vi "Trim_log.vi"(8 "error in (no error)":errorcluster, 9 "% to trim":i32=75 caption="% to trim (75)", 11 "Log File Refnum":refnum<file>) -> (0 "error out":errorcluster, 3 "Log File Refnum (out)":refnum<file>)   [LabVIEW 2010, in "lib1299.lvlib"]
uses:
  lib1299.lvlib
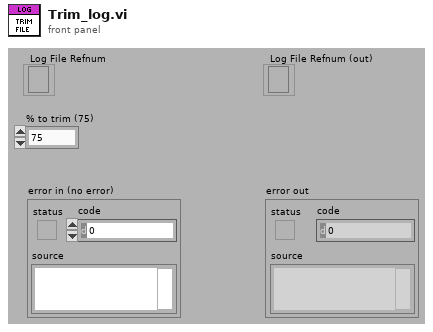
[diagram p1: front panel]
types:
  T1 = enum16{"open", "replace", "create", "open or create", "replace or create", "replace or create with confirmation"}
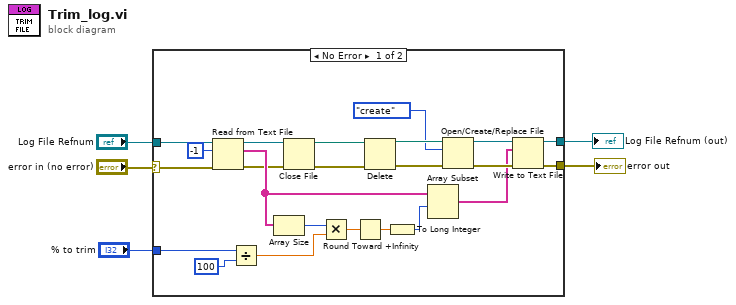
[diagram p0: block diagram]
diagram:
  n1 = case shown="No Error" "error in (no error)" {
    selector: "error in (no error)" -> [w7 w29]
    tunnel: "% to trim" -> [w25 _]
    tunnel: "Log File Refnum" -> [w19 w30]
    tunnel: [w8 w30] -> w3
    tunnel: [w6 w29] -> w1
    frame No Error {
      n2 = Read from Text File(file (use dialog)=w19, count=-1, error in=w7) -> (refnum out=w17:refnum<file>, text=w24:string[], error out=w18:errorcluster)  [unwired: 1 in, 1 out]
      n3 = Divide(x=w25, y=100 ("x")) -> (x/y=w21:dbl)
      n4 = Array Size(array=w24) -> (size(s)=w23:i32)
      n5 = Close File(refnum=w17, error in=w18) -> (path=w16:path, error out=w15:errorcluster)
      n6 = Multiply(x=w23, y=w21) -> (x*y=w26:dbl)
      n7 = Round Toward +Infinity(x=w26) -> (ceil(x): smallest int >= x=w27:dbl)
      n8 = Delete(path (use dialog)=w16, error in=w15) -> (deleted path=w13:path, error out=w14:errorcluster)  [unwired: 3 in, 1 out]
      n9 = To Long Integer(number=w27) -> (32bit integer=w28:i32)
      n10 = Array Subset(array=w24, index=w28) -> (w9:string[])  [unwired: 1 in]
      n11 = Open/Create/Replace File(file path (use dialog)=w13, error in=w14, operation (0:open)=T1."create") -> (refnum out=w11:refnum<file>, error out=w10:errorcluster)  [unwired: 3 in, 1 out]
      n12 = Write to Text File(file (use dialog)=w11, text=w9, error in=w10) -> (refnum out=w8:refnum<file>, error out=w6:errorcluster)  [unwired: 1 in, 1 out]
    }
    frame Error {
    }
  }
  "Log File Refnum (out)" <- w3
  "error out" <- w1
